vi "Disable Laser.vi"(8 "error in (no error)":errorcluster, 11 "VISA Refnum in":refnum<visa-resource-name>) -> (0 "error out":errorcluster, 3 "VISA Refnum out":refnum<visa-resource-name>)   [LabVIEW 2016]
doc: "This VI deactivates the URG-04LX's laser."
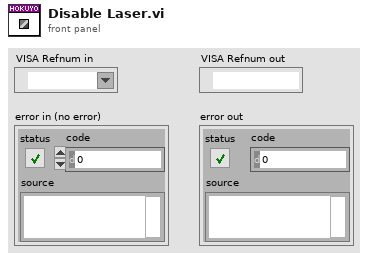
[diagram p1: front panel]
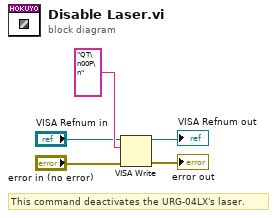
[diagram p0: block diagram]
diagram:
  # "This command deactivates the URG-04LX's laser."
  n1 = VISA Write(VISA resource name="VISA Refnum in", write buffer="QT\n00P\n", error in (no error)="error in (no error)") -> (VISA resource name out=→"VISA Refnum out":refnum<visa-resource-name>, error out=→"error out":errorcluster)  [unwired: 1 out]
